vi "Get Alliance.vi"() -> (3 "Alliance":T1)   [LabVIEW 2025]
uses:
  <vilib>/Rock Robotics/WPI/DriverStation/WPI_DriverStationAllianceInfo.ctl
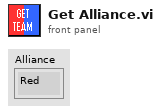
[diagram p1: front panel]
types:
  T1 = typedef "WPI_DriverStationAllianceInfo.ctl" = enum16{"Red", "Blue", "Invalid"}
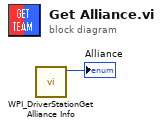
[diagram p0: block diagram]
diagram:
  n1 = call <vilib>:"WPI_DriverStationGet Alliance Info.vi"() -> ("Alliance"=→"Alliance":T1)  [unwired: 6 in, 5 out]
